vi "Pre Launch Init.vi"(11 "RandomNumberModel in":refnum<class "RandomNumberModel.lvclass">) -> (0 "error out":errorcluster, 3 "RandomNumberModel out":refnum<class "RandomNumberModel.lvclass">)   [LabVIEW 2017, in "RandomNumberModel.lvlib" / "RandomNumberModel.lvclass"]
doc: "(<B>Filename</B>: Actor Framework.lvlib:Actor.lvclass:Pre Launch Init.vi)\n\nDefines behavior that occurs after the Launch Nested Actor method is invoked but before the actor's Actor Core method begins running.\n\nBy default, this method does nothing. A descendant class may override it to define behavior.MVA Framework 1.7.0.33\nEthan Stern - Composed Systems\nCopyright (c) 2018, Composed Systems"
uses:
  <vilib>/gpm_packages/@cs/example/Dynamic Viewables/SequenceSteps/RandomNumberModel/RandomNumberModel.lvclass
  C:/Program Files/National Instruments/LabVIEW 2017/vi.lib/gpm_packages/@cs/mva-core/Source/IModel/IModel/IModel.lvclass
  C:/Program Files/National Instruments/LabVIEW 2017/vi.lib/ActorFramework/Actor/Actor.lvclass
  <vilib>/gpm_packages/@cs/mva-core/Source/IObserver/IObserver/IObserver.lvclass/IObserver.ctl
  <vilib>/gpm_packages/@cs/mva-core/Source/IModel/IModel/IModel.lvclass/IModel.ctl
  <vilib>/gpm_packages/@cs/mva-core/Source/IMediator/PublishRequest/PublishRequest.lvclass/PublishRequest.ctl
  <vilib>/gpm_packages/@cs/mva-core/Source/IMediator/IMediator Messages/Publish Msg/Publish Msg.lvclass/Publish Msg.ctl
  <vilib>/gpm_packages/@cs/actor-framework-messages/Source/RoundTripMessage/RoundTripMessage.lvclass/RoundTripMessage.ctl
  <vilib>/ActorFramework/Message Enqueuer/Message Enqueuer.lvclass/Message Enqueuer.ctl
  <vilib>/ActorFramework/Actor/Actor.lvclass/Actor.ctl
  <vilib>/gpm_packages/@cs/example/Dynamic Viewables/SequenceSteps/RandomNumberModel/RandomNumberModel.lvclass/RandomNumberModel.ctl
  <vilib>/ActorFramework/Message Enqueuer/Init from Existing Queue.vi
  <vilib>/ActorFramework/Message Enqueuer/Enqueue.vi
  <vilib>/gpm_packages/@cs/mva-core/Source/IMediator/IMediator Messages/Publish Msg/Send Pre-Addressed Publish.vi
  <vilib>/gpm_packages/@cs/mva-core/Source/IObserver/IObserver/Read Unique ID.vi
  <vilib>/gpm_packages/@cs/mva-core/Source/IMediator/PublishRequest/Pack Publish Request.vi
  <vilib>/gpm_packages/@cs/actor-framework-messages/Source/RoundTripMessage/Return Round-Trip Message.vi
  <vilib>/gpm_packages/@cs/mva-core/Source/IModel/IModel/IModel.lvclass
  C:/Program Files/National Instruments/LabVIEW 2017/vi.lib/gpm_packages/@cs/mva-core/Source/IObserver/IObserver/IObserver.lvclass
  <vilib>/gpm_packages/@cs/mva-core/Source/IMediator/IMediator Messages/Publish Msg/Publish Msg.lvclass
  C:/Program Files/National Instruments/LabVIEW 2017/vi.lib/gpm_packages/@cs/actor-framework-messages/Source/RoundTripMessage/RoundTripMessage.lvclass
  <vilib>/gpm_packages/@cs/actor-framework-messages/Source/RoundTripMessage/RoundTripMessage.lvclass
  C:/Program Files/National Instruments/LabVIEW 2017/vi.lib/ActorFramework/Message/Message.lvclass
  <vilib>/gpm_packages/@cs/example/Dynamic Viewables/SequenceSteps/RandomNumberModel Messages/GenerateRandomNumber Msg/GenerateRandomNumber Msg.lvclass
  <vilib>/ActorFramework/Message Priority Queue/Priority Enqueue.vi
  <vilib>/Utility/error.llb/Error Cluster From Error Code.vi
  <vilib>/ActorFramework/Message Enqueuer/Message Enqueuer.lvclass
  <vilib>/gpm_packages/@cs/mva-core/Source/IMediator/PublishRequest/PublishRequest.lvclass
  <vilib>/ActorFramework/Actor/Actor.lvclass
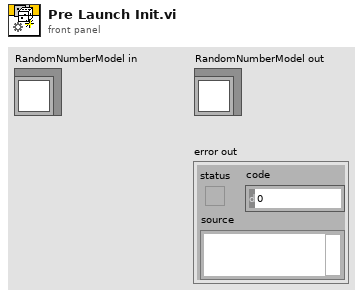
[diagram p1: front panel]
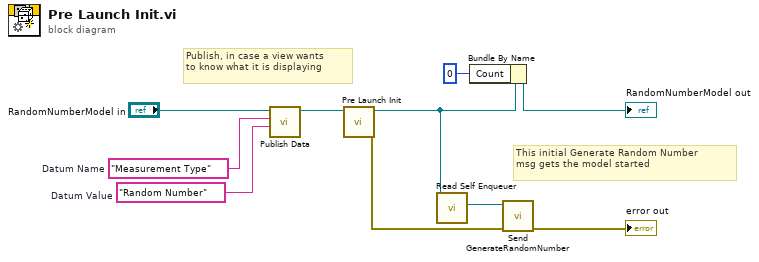
[diagram p0: block diagram]
diagram:
  w1 = "Random Number"  # Datum Value
  w2 = "Measurement Type"  # Datum Name
  # "Publish, in case a view wants\nto know what it is displaying"
  # "This initial Generate Random Number\nmsg gets the model started"
  n1 = call <vilib>:"Publish Data.vi"("Data to Publish"=w1, "Datum Name"=w2, "IModel in"="RandomNumberModel in") -> ("IModel out"=w3:refnum<class "RandomNumberModel.lvclass">)  [unwired: 7 in, 1 out]
  n2 = call-parent "Pre Launch Init.vi"("IModel in"=w3) -> ("error out"=w7:errorcluster, "IModel out"=w9:refnum<class "RandomNumberModel.lvclass">)  [unwired: 9 in]
  n3 = call <vilib>:"Read Self Enqueuer.vi"("Actor"=w9) -> ("Self Enqueuer"=w8:refnum<class "Message Enqueuer.lvclass">)  [unwired: 10 in]
  n4 = Bundle By Name(cluster=w9, "Count"=0 ("Numbers Generated")) -> (→"RandomNumberModel out":refnum<class "RandomNumberModel.lvclass">)
  n5 = call <vilib>:"Send GenerateRandomNumber.vi"("error in (no error)"=w7, "Message Enqueuer"=w8) -> ("error out"=→"error out":errorcluster)  [unwired: 8 in, 1 out]
